vi "CheckCreateFile.vi"(8 "Error In":errorcluster, 10 "Folder":string, 11 "Image Name":string) -> (0 "Error Out":errorcluster, 3 "File Path":path)   [LabVIEW 2015]
doc: "VI Checks for a folder in the application\ndirectory. If it doesn't existe, the VI\ncreates the folder and returns the path of the\nimage that is being saved there. \n\nAlso checks to see if image already exists. If so, increments\nthe last number character before .jpg and saves the new image\nin the directory above."
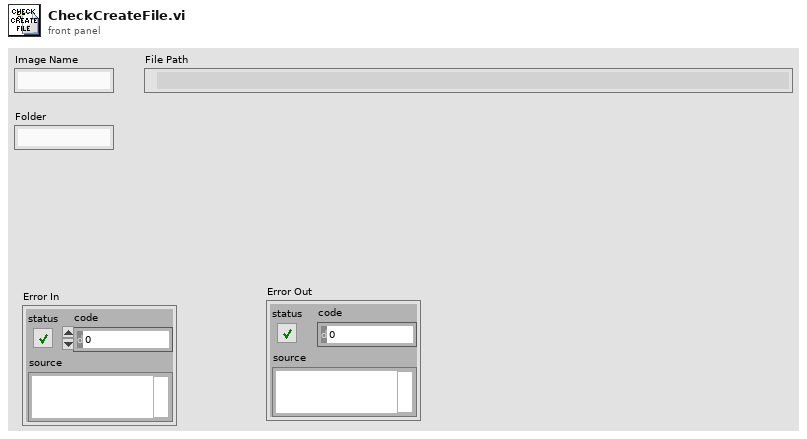
[diagram p1: front panel]
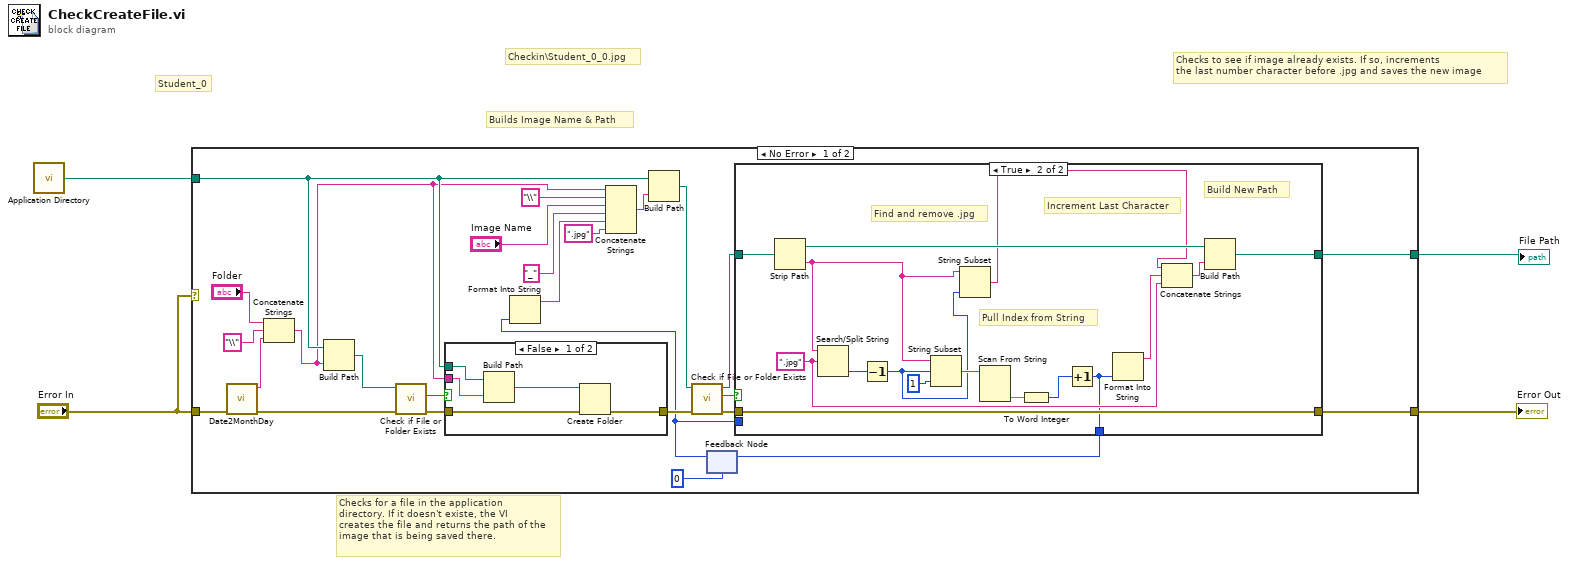
[diagram p0: block diagram]
diagram:
  # "Checkin\\Student_0_0.jpg"
  # "Student_0"
  # "Builds Image Name & Path"
  # "Checks to see if image already exists. If so, increments\nthe last number character before .jpg and saves the new image"
  # "Checks for a file in the application\ndirectory. If it doesn't existe, the VI\ncreates the file and returns the path of the\nimage that is being saved there."
  n1 = call <vilib>:"Application Directory.vi"() -> ("Application Directory"=w1:path)
  n2 = case shown="No Error" "Error In" {
    tunnel: "Error In" -> [w9 w57]
    tunnel: [w17 w57] -> w4
    tunnel: [w15 w56] -> w2
    tunnel: w1 -> [w14 w56]
    frame No Error {
      n3 = call "Date2MonthDay.vi"("Error In"=w9) -> ("Error Out"=w10:errorcluster, "MonthDay"=w6:string)  [unwired: 9 in]
      n4 = Concatenate Strings("Folder", "\\" ("string"), w6) -> (w5:string)
      n5 = Build Path(base path=w14, name or relative path=w5) -> (appended path=w29:path)
      n6 = call <vilib>:"Check if File or Folder Exists.vi"("error in (no error)"=w10, "path"=w29) -> ("error out"=w30:errorcluster, "file or folder exists?"=w28:bool)  [unwired: 7 in, 1 out]
      n7 = case shown="False" w28 {
        tunnel: w14 -> [w54 _]
        tunnel: w5 -> [w52 _]
        tunnel: [w51 w55] -> w18
        tunnel: w30 -> [w50 w55]
        frame False {
          n8 = Build Path(base path=w54, name or relative path=w52) -> (appended path=w53:path)
          n9 = Create Folder(path (use dialog)=w53, error in=w50) -> (error out=w51:errorcluster)  [unwired: 1 in, 2 out]
        }
        frame True {
        }
      }
      n10 = feedback #1(0) -> (w11:i32)
      n11 = Format Into String(w11) -> (resulting string=w22:string)  [unwired: 3 in, 1 out]
      n12 = Concatenate Strings(w5, "\\" ("string"), "Image Name", "_" ("string"), w22, ".jpg" ("string")) -> (w26:string)
      n13 = Build Path(base path=w14, name or relative path=w26) -> (appended path=w21:path)
      n14 = call <vilib>:"Check if File or Folder Exists.vi"("error in (no error)"=w18, "path"=w21) -> ("error out"=w16:errorcluster, "file or folder exists?"=w20:bool, "dup path"=w19:path)  [unwired: 7 in]
      n15 = case shown="True" w20 {
        tunnel: w19 -> [w33 w49]
        tunnel: [w33 w40] -> w15
        tunnel: [w32 w38] -> w17
        tunnel: w16 -> [w32 w38]
        tunnel: [w31 w34] -> w13
        tunnel: w11 -> [w31 _]
        frame False {
        }
        frame True {
          w42 = ".jpg" ("search string/char (-)")
          # "Build New Path"
          # "Increment Last Character"
          # "Find and remove .jpg"
          # "Pull Index from String"
          n16 = Strip Path(path=w49) -> (stripped path=w43:path, name=w37:string)
          n17 = Search/Split String(string=w37, search string/char (-)=w42) -> (offset of match=w47:i32)  [unwired: 1 in, 2 out]
          n18 = Decrement(x=w47) -> (x-1=w36:i32)
          n19 = String Subset(string=w37, offset (0)=w36, length (rest)=1 ("length (rest)")) -> (substring=w45:string)
          n20 = String Subset(string=w37, length (rest)=w36) -> (substring=w35:string)  [unwired: 1 in]
          n21 = Scan From String(input string=w45) -> (output 1=w46:dbl)  [unwired: 4 in, 3 out]
          n22 = To Word Integer(number=w46) -> (16bit integer=w39:i16)
          n23 = Increment(x=w39) -> (x+1=w34:i16)
          n24 = Format Into String(w34) -> (resulting string=w44:string)  [unwired: 3 in, 1 out]
          n25 = Concatenate Strings(w35, w44, w42) -> (w41:string)
          n26 = Build Path(base path=w43, name or relative path=w41) -> (appended path=w40:path)
        }
      }
      n27 = feedback-in #1(w13) -> ()
    }
    frame Error {
    }
  }
  "Error Out" <- w4
  "File Path" <- w2
